vi "commandApplyAberrationByForces.vi"(8 "error in (no error)":errorcluster, 10 "CommandApplyAberrationByForces in":T1, 11 "M1M3SAL in":refnum<class "M1M3SAL.lvclass">) -> (0 "error out":errorcluster, 2 "CommandApplyAberrationByForces out":T1, 3 "M1M3SAL out":refnum<class "M1M3SAL.lvclass">)   [LabVIEW 2016, in "M1M3SupportCommunicator.lvlib" / "M1M3SAL.lvclass"]
uses:
  M1M3SAL.lvclass
  DataTypes/Topics/CommandApplyAberrationByForces.ctl
  DataTypes/Topics/Parts/CommandId.ctl
  DataTypes/MessageHeader.ctl
  DataTypes/MessageTypes.ctl
  DataTypes/MessageTopics.ctl
  Common_RT_Utilities/U8ArrayBuilderAutoIndexing/U8ArrayBuilderAutoIndexing.lvclass
  M1M3SupportCommunicator.lvlib
  DataTypes/Topics/M1M3SupportTopics.lvlib
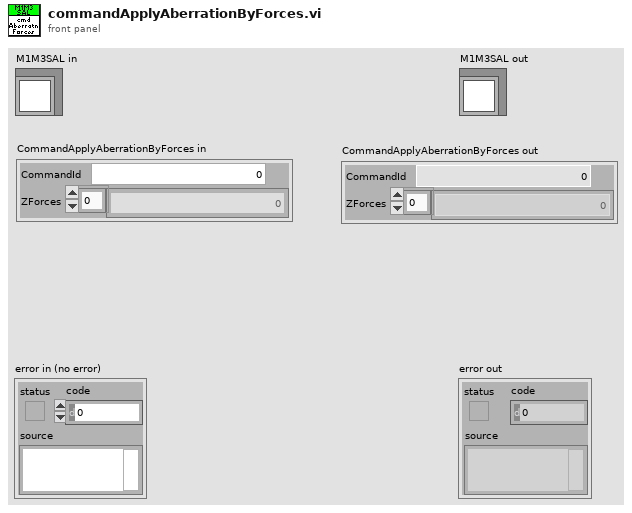
[diagram p1: front panel]
types:
  T1 = typedef "M1M3SupportTopics.lvlib/CommandApplyAberrationByForces.ctl" = cluster{"CommandId":T2, "ZForces":dbl[]}
  T2 = typedef "M1M3SupportTopics.lvlib/CommandId.ctl" = i32
  T3 = typedef "M1M3SupportCommunicator.lvlib/MessageHeader.ctl" = cluster{"Type":T4, "Topic":T5, "Size":i32}
  T4 = typedef "M1M3SupportCommunicator.lvlib/MessageTypes.ctl" = enum8{"None", "PutSample", "GetNextSample", "LogEvent", "GetEvent", "IssueCommand", "CommandId", "WaitForCompletion", "AcceptCommand", "AckCommand"}
  T5 = typedef "M1M3SupportCommunicator.lvlib/MessageTopics.ctl" = enum8{"None", "ForceActuatorData", "MirrorForceData", "HardpointData", "AirData", "DynamicData", "FPGAData", "IMSData", "ForceActuatorStatus", "ElevationData", "HardpointStatus", "HardpointActuatorChase", "AirStatus", "ForceActuatorSafetyChecks", "ForceActuatorTest", "ActuatorBroadcastCounter", "StatusChecks", "CellChecks", "HardpointActuatorBreakaway", "RaiseMirrorComplete", "ILCCommunication", "ElevationAngleChecks", "DetailedState", "ServoLoops", "ForceActuatorInfo", "LowerMirrorComplete", "HardpointActuatorInfo", "SettingsApplied", "ErrorCode", "StartupChecks", "SummaryState", "SettingVersions", "ActuatorTestStatus", "AppliedSettingsMatchStart", "Enable", "EnterMaintenance", "Standby", "AbortLowerM1M3", "ApplyAberrationByForces", "ApplyAOSCorrectionByBendingModes", "ClearAOSCorrection", "Start", "RaiseM1M3", "TestForceActuator", "LowerM1M3", "ApplyAOSCorrectionByForces", "Disable", "ApplyAberationByBendingMode", "TestHardpoint", "ManipulateM1M3", "ClearAberration", "Exit", "TestAir", "AbortRaiseM1M3", "MoveHardpointActuators", "ExitMaintenance", "Shutdown"}
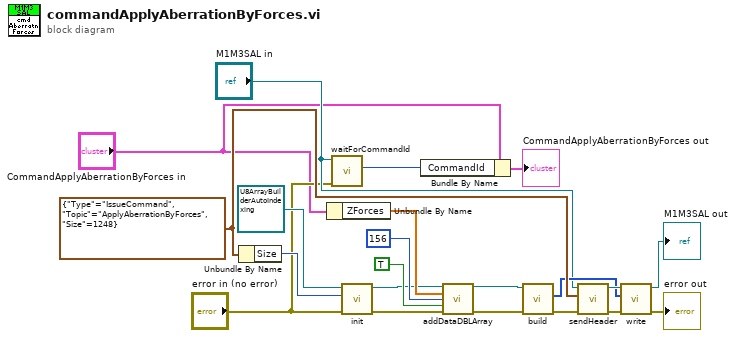
[diagram p0: block diagram]
diagram:
  w20 = T3 {"Type"=enum."IssueCommand", "Topic"=enum."ApplyAberrationByForces", "Size"=1248} ("MessageHeader")
  n1 = Unbundle By Name(w20) -> ("Size"=w19:i32)
  n2 = Unbundle By Name("CommandApplyAberrationByForces in") -> ("ZForces"=w7:dbl[])
  n3 = call "waitForCommandId.vi"("error in (no error)"="error in (no error)", "M1M3SAL in"="M1M3SAL in") -> ("CommandId"=w14:T2)  [unwired: 7 in, 2 out]
  n4 = call "init.vi"("error in (no error)"="error in (no error)", "Size"=w19, "U8ArrayBuilderAutoIndexing in"=refnum<class "U8ArrayBuilderAutoIndexing.lvclass"> refnum ("RTUtilities.lvlib:U8ArrayBuilderAutoIndexing.lvclass")) -> ("error out"=w5:errorcluster, "U8ArrayBuilderAutoIndexing out"=w6:refnum<class "U8ArrayBuilderAutoIndexing.lvclass">)  [unwired: 7 in]
  n5 = Bundle By Name(cluster="CommandApplyAberrationByForces in", "CommandId"=w14) -> (→"CommandApplyAberrationByForces out":T1)
  n6 = call "addDataDBLArray.vi"("U8ArrayBuilderAutoIndexing in"=w6, "Data"=w7, "Length"=156, "OverrideSwapBytes"=TRUE, "error in (no error)"=w5) -> ("U8ArrayBuilderAutoIndexing out"=w3:refnum<class "U8ArrayBuilderAutoIndexing.lvclass">, "error out"=w4:errorcluster)  [unwired: 9 in]
  n7 = call "build.vi"("error in (no error)"=w4, "U8ArrayBuilderAutoIndexing in"=w3) -> ("error out"=w16:errorcluster, "Array"=w17:u8[])  [unwired: 7 in, 1 out]
  n8 = call "sendHeader.vi"("error in (no error)"=w16, "MessageHeader"=w20, "M1M3SAL in"="M1M3SAL in") -> ("error out"=w15:errorcluster, "M1M3SAL out"=w18:refnum<class "M1M3SAL.lvclass">)  [unwired: 7 in]
  n9 = call "write.vi"("error in (no error)"=w15, "Data"=w17, "M1M3SAL in"=w18) -> ("error out"=→"error out":errorcluster, "M1M3SAL out"=→"M1M3SAL out":refnum<class "M1M3SAL.lvclass">)  [unwired: 7 in]
